vi "PrimedStateFGV.vi"(3 "Enum":enum16{"Set Values", "Set Time", "Get Values"}(ring), 7 "LastValve_write":i32) -> (8 "LastValve_read":i32, 15 "Time_read":timestamp)   [LabVIEW 2019]
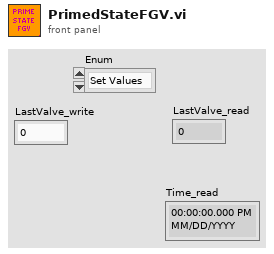
[diagram p1: front panel]
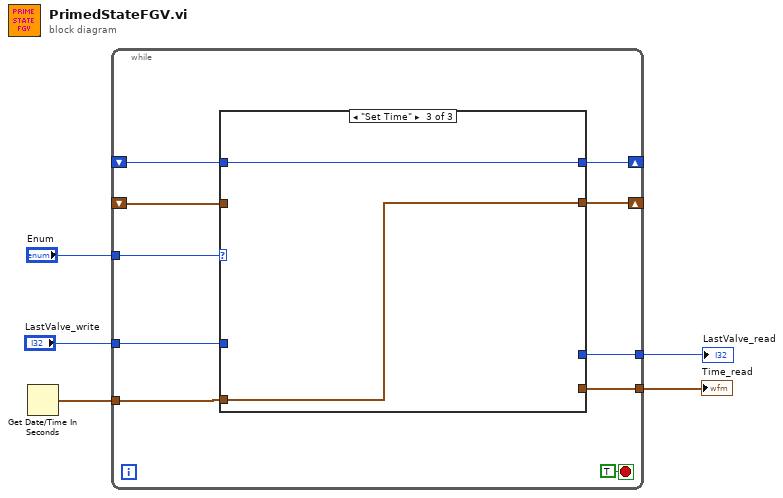
[diagram p0: block diagram]
diagram:
  n1 = Get Date/Time In Seconds() -> (seconds since 1Jan1904=w1:timestamp)
  n2 = while {
    tunnel: "Enum" -> [w15]
    shift-right: [w13] -> _
    shift-left: _ -> [w14]
    tunnel: [w12] -> w3
    tunnel: "LastValve_write" -> [w10]
    tunnel: w1 -> [w9]
    shift-right: [w8] -> _
    shift-left: _ -> [w7]
    tunnel: [w6] -> w2
    stop <- TRUE ("stop") stop-if-true
    n3 = case shown="\"Set Time\"" w15 {
      tunnel: w10 -> [w17 _ _]
      tunnel: w14 -> [_ w19 w20]
      tunnel: [w17 w19 w20] -> w13
      tunnel: [_ w19 _] -> w12
      tunnel: w9 -> [w16 _ w21]
      tunnel: [w16 w18 w21] -> w8
      tunnel: w7 -> [_ w18 _]
      tunnel: [_ w18 _] -> w6
      frame "Set Values", Default {
      }
      frame "Get Values" {
      }
      frame "Set Time" {
      }
    }
  }
  "LastValve_read" <- w3
  "Time_read" <- w2
